vi "StopMovement.vi"(8 "error in (no error)":errorcluster, 10 "AxisNumber":u8, 11 "CS++Motor in":refnum<class "CS++Motor.lvclass">) -> (0 "error out":errorcluster, 3 "CS++Motor out":refnum<class "CS++Motor.lvclass">)   [LabVIEW 2015, in "CS++Motor.lvlib" / "CS++Motor.lvclass"]
doc: "Stops the movement of an axis."
uses:
  CS++Motor.lvclass
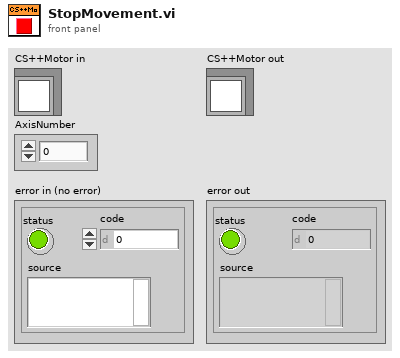
[diagram p1: front panel]
types:
  T1 = enum16{"NormalMovement", "ReferenceMovement", "StopMovement"}
  T2 = cluster{"MovementType":enum16{"NormalMovement", "ReferenceMovement", "StopMovement"}, "SetPosition":dbl, "Relative?":bool}
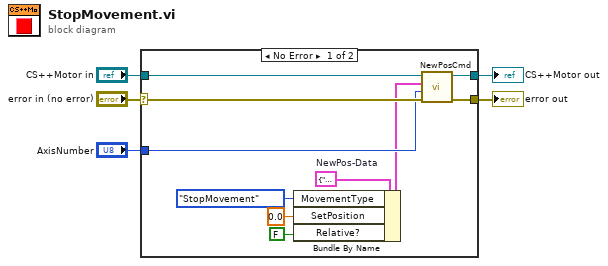
[diagram p0: block diagram]
diagram:
  n1 = case shown="No Error" "error in (no error)" {
    selector: "error in (no error)" -> [w11 w17]
    tunnel: [w10 w17] -> w4
    tunnel: [w8 w16] -> w5
    tunnel: "CS++Motor in" -> [w9 w16]
    tunnel: "AxisNumber" -> [w7 _]
    frame No Error {
      w15 = T2 {"MovementType"=enum."NormalMovement", "SetPosition"=0.0, "Relative?"=FALSE}  # NewPos-Data
      n2 = Bundle By Name(cluster=w15, "MovementType"=T1."StopMovement", "SetPosition"=0.0, "Relative?"=FALSE) -> (w6:T2)
      n3 = call "NewPosCmd.vi"("error in (no error)"=w11, "AxisNumber"=w7, "NewPos-Data"=w6, "CS++Motor in"=w9) -> ("error out"=w10:errorcluster, "CS++Motor out"=w8:refnum<class "CS++Motor.lvclass">)  [unwired: 6 in]
    }
    frame Error {
    }
  }
  "error out" <- w4
  "CS++Motor out" <- w5
